vi "Create Example App Properties.vi"(8 "error in (no error)":errorcluster, 11 "Acrobat Template in":refnum<class "Example Application.lvclass">) -> (0 "error out":errorcluster, 3 "Acrobat Template out":refnum<class "Example Application.lvclass">)   [LabVIEW 2015, in "Example Application.lvlib" / "Example Application.lvclass"]
uses:
  Example Application.lvclass
  Properties/Example App Properties.lvclass
  Example Application.lvclass/Example Application.ctl
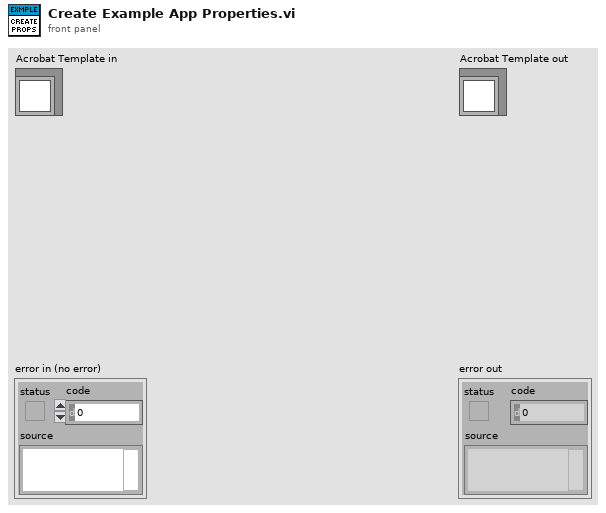
[diagram p1: front panel]
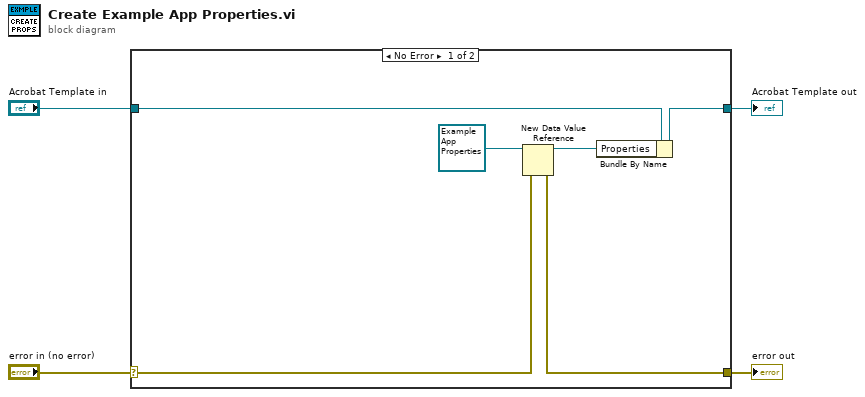
[diagram p0: block diagram]
diagram:
  n1 = case shown="No Error" "error in (no error)" {
    selector: "error in (no error)" -> [w8 w12]
    tunnel: [w7 w12] -> w3
    tunnel: [w9 w11] -> w1
    tunnel: "Acrobat Template in" -> [w10 w11]
    frame No Error {
      n2 = New Data Value Reference(data value=refnum<class "Example App Properties.lvclass"> refnum ("Acrobat Object Template.lvlib:Template Properties.lvclass"), error in=w8) -> (data value reference=w6:refnum<data-value>, error out=w7:errorcluster)
      n3 = Bundle By Name(cluster=w10, "Properties"=w6) -> (w9:refnum<class "Example Application.lvclass">)
    }
    frame Error {
    }
  }
  "error out" <- w3
  "Acrobat Template out" <- w1
